vi "EEG - Fast Fourier Transform.vi"() -> ()   [LabVIEW 2013]
uses:
  <vilib>/addons/Biomedical/Biosignal Measurements/EEG/subVIs/bmt_EEG FFT Settings.ctl
  <vilib>/addons/Biomedical/Biosignal Measurements/EEG/subVIs/bmt_EEG Frequency Bands.ctl
  <vilib>/addons/Biomedical/Controls/Biosignal/Biosignal Spectrum/Biosignal Spectrum.xctl
  <vilib>/addons/Biomedical/Biosignal Measurements/EEG/EEG FFT Spectrum (Array).vi
  <vilib>/addons/Biomedical/NI_BMTK_Measurements.lvlib
  <vilib>/addons/Biomedical/NI_BMTK_Controls.lvlib
panel:
  in  "Frekvencija odabiranja":dbl=1.0
  out "Signal pre analize":waveform(dbl)[](graph)
  out "Lokacija sacuvanog fajla na racunaru":path
  out "FFT spektar":cluster{"f0":dbl, "df":dbl, "S(f)":dbl[]}(xcontrol)
  out "Delta Snaga":dbl format="%#_2f uV^2"
  out "Teta Snaga":dbl format="%#_2f uV^2"
  out "Alfa Snaga":dbl format="%#_2f uV^2"
  out "Delta [%]":dbl format="%#_2f %"
  out "Teta [%]":dbl format="%#_2f %"
  out "Alfa [%]":dbl format="%#_2f %"
  out "Beta Snaga":dbl format="%#_2f uV^2"
  out "Beta [%]":dbl format="%#_2f %"
  in  "FFT podesavanja":T1={"podesavanje prozora"={"vrsta"=1, "duzina"=1024, "preklapanje [%]"=50.0}, "frekventni opsezi"={"delta high"=4.0, "delta low"=0.5, "theta high"=7.5, "theta low"=4.0, "alpha high"=13.0, "alpha low"=8.0, "beta high"=26.0, "beta low"=14.0}, "dB on? (F)"=FALSE, "frekventni binovi"=1024} {"podesavanje prozora"."vrsta" items=["None ", "Hanning", "Hamming", "Blackman-Harris", "Exact Blackman", "Blackman", "Flat Top", "4 Term B-Harris ", "7 Term B-Harris", "Low Sidelobe"]}
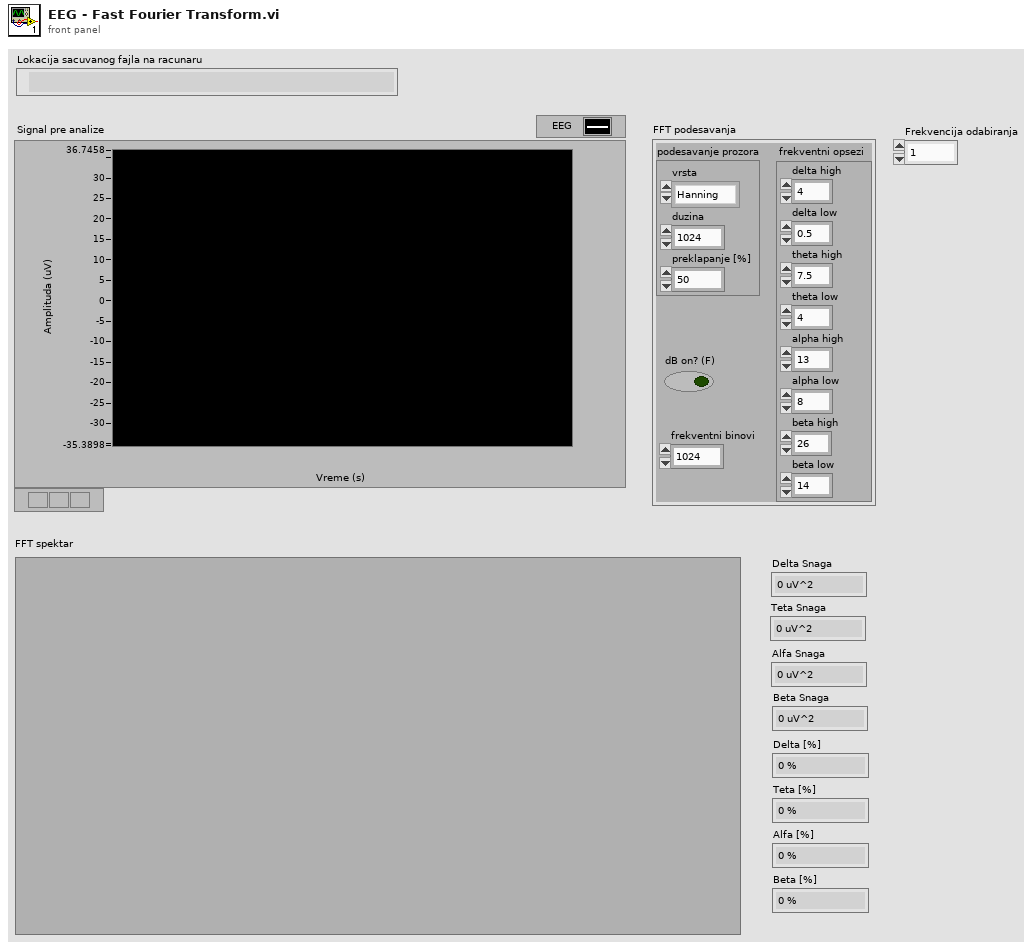
[diagram p1: front panel]
types:
  T1 = typedef "NI_BMTK_Measurements.lvlib/bmt_EEG FFT Settings.ctl" = cluster{"podesavanje prozora":cluster{"vrsta":u16, "duzina":i32, "preklapanje [%]":dbl}, "frekventni opsezi":T2, "dB on? (F)":bool, "frekventni binovi":i32}
  T2 = typedef "NI_BMTK_Measurements.lvlib/bmt_EEG Frequency Bands.ctl" = cluster{"delta high":dbl, "delta low":dbl, "theta high":dbl, "theta low":dbl, "alpha high":dbl, "alpha low":dbl, "beta high":dbl, "beta low":dbl}
  T3 = enum16{"open", "open or create", "create or replace", "create", "open (read-only)"}
  T4 = typedef "NI_BMTK_Measurements.lvlib/bmt_EEG Frequency-domain Measures.ctl" = cluster{"delta power":dbl, "theta power":dbl, "alpha power":dbl, "beta power":dbl, "delta [%]":dbl, "theta [%]":dbl, "alpha [%]":dbl, "beta [%]":dbl}
  T5 = enum16{"open", "replace", "create", "open or create", "replace or create", "replace or create with confirmation"}
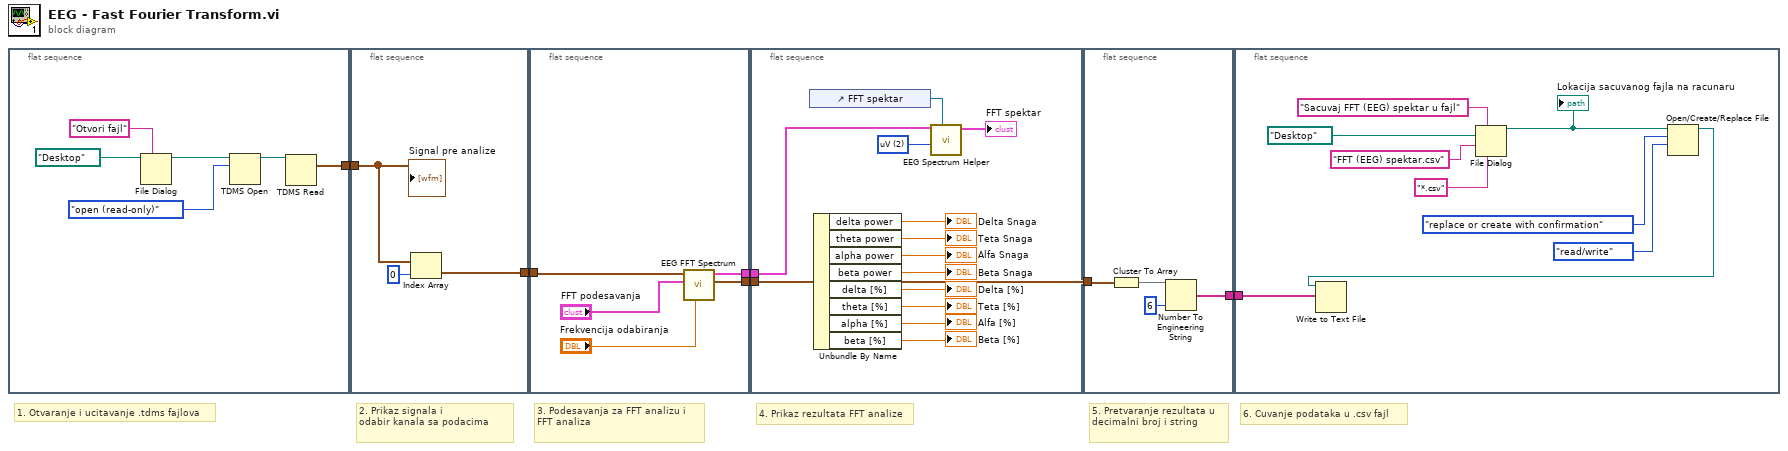
[diagram p0: block diagram]
diagram:
  # "6. Cuvanje podataka u .csv fajl"
  # "5. Pretvaranje rezultata u decimalni broj i string"
  # "4. Prikaz rezultata FFT analize"
  # "3. Podesavanja za FFT analizu i FFT analiza"
  # "2. Prikaz signala i \nodabir kanala sa podacima"
  # "1. Otvaranje i ucitavanje .tdms fajlova"
  n1 = flat-sequence {
    tunnel: [w7] -> w2
    frame #0 {
      n2 = File Dialog(7:"Otvori fajl" ("prompt"), 11:path "/Desktop" ("start path")) -> (3:w9:path)  [unwired: 2 in, 6 out]
      n3 = TDMS Open(10:T3."open (read-only)" ("operation (0:open)"), 11:w9) -> (3:w10:refnum<k34>)  [unwired: 5 in, 1 out]
      n4 = TDMS Read(0:w10) -> (10:w7:waveform(dbl)[])  [unwired: 7 in, 5 out]
    }
  }
  n5 = flat-sequence {
    tunnel: w2 -> [w14]
    tunnel: [w12] -> w1
    frame #0 {
      n6 = Index Array(array=w14, index=0) -> (element=w12:waveform(dbl))
      "Signal pre analize" <- w14
    }
  }
  n7 = flat-sequence {
    tunnel: [w18] -> w5
    tunnel: [w17] -> w3
    tunnel: w1 -> [w16]
    frame #0 {
      n8 = call-poly <vilib>:"EEG FFT Spectrum.vi"("sampling rate"="Frekvencija odabiranja", "FFT settings"="FFT podesavanja", "EEG"=w16) -> ("frequency measurements"=w18:T4, "FFT spectrum"=w17:cluster{"f0":dbl, "df":dbl, "S(f)":dbl[]})  [unwired: 6 in, 1 out]
    }
  }
  n9 = flat-sequence {
    tunnel: w5 -> [w21]
    tunnel: w3 -> [w20]
    frame #0 {
      w32 = u16 2 items=["V", "mV", "uV"] ("RR unit")
      n10 = control-ref of="FFT spektar"() -> (w31:refnum<vi>)
      n11 = Unbundle By Name(w21) -> ("delta power"=→"Delta Snaga":dbl, "theta power"=→"Teta Snaga":dbl, "alpha power"=→"Alfa Snaga":dbl, "beta power"=→"Beta Snaga":dbl, "delta [%]"=→"Delta [%]":dbl, "theta [%]"=→"Teta [%]":dbl, "alpha [%]"=→"Alfa [%]":dbl, "beta [%]"=→"Beta [%]":dbl)
      n12 = call <vilib>:"EEG Spectrum Helper.vi"("EEG spectrum"=w31, "EEG unit"=w32, "spectrum in"=w20) -> ("spectrum out"=→"FFT spektar":cluster{"f0":dbl, "df":dbl, "S(f)":dbl[]})  [unwired: 7 in, 1 out]
    }
  }
  n13 = flat-sequence {
    tunnel: w5 -> [w36]
    tunnel: [w35] -> w4
    frame #0 {
      n14 = Cluster To Array(cluster=w36) -> (array=w34:dbl[])
      n15 = Number To Engineering String(2:i16 6 ("precision (6)"), 4:w34) -> (0:w35:string[])  [unwired: 2 in]
    }
  }
  n16 = flat-sequence {
    tunnel: w4 -> [w37]
    frame #0 {
      n17 = File Dialog(6:"*.csv" ("pattern (all files)"), 7:"Sacuvaj FFT (EEG) spektar u fajl" ("prompt"), 9:"FFT (EEG) spektar.csv" ("default name"), 11:path "/Desktop" ("start path")) -> (3:w40:path)  [unwired: 1 in, 5 out]
      "Lokacija sacuvanog fajla na racunaru" <- w40
      n18 = Open/Create/Replace File(file path (use dialog)=w40, operation (0:open)=T5."replace or create with confirmation", access (0:read/write)=enum16{"read/write", "read-only", "write-only"}."read/write") -> (refnum out=w38:refnum<file>)  [unwired: 3 in, 2 out]
      n19 = Write to Text File(file (use dialog)=w38, text=w37) -> ()  [unwired: 2 in, 3 out]
    }
  }
